vi "导入Excel.vi"(8 "error in (no error)":errorcluster) -> (0 "error out":errorcluster, 3 "data":string[][](array[string]))   [LabVIEW 2016, in "Alarm interface.lvlib"]
uses:
  Alarm interface.lvlib
  <vilib>/addons/_office/excel.llb/Excel Get Data ([str]).vi
  <vilib>/regexp/Match Regular Expression.xnode
  <vilib>/Utility/NIReport.llb/NI_report.lvclass
  <vilib>/Utility/NIReport.llb/Excel/NI_Excel.lvclass
  <vilib>/addons/_office/NI_ReportGenerationToolkit.lvlib
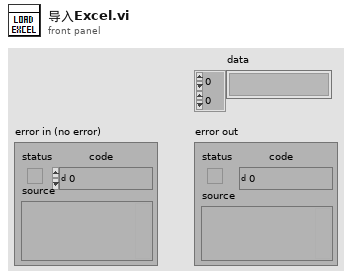
[diagram p1: front panel]
types:
  T1 = enum16{"Standard Report", "HTML", "Word", "Excel"}
  T2 = enum16{"maximized", "minimized", "normal", "no change"}
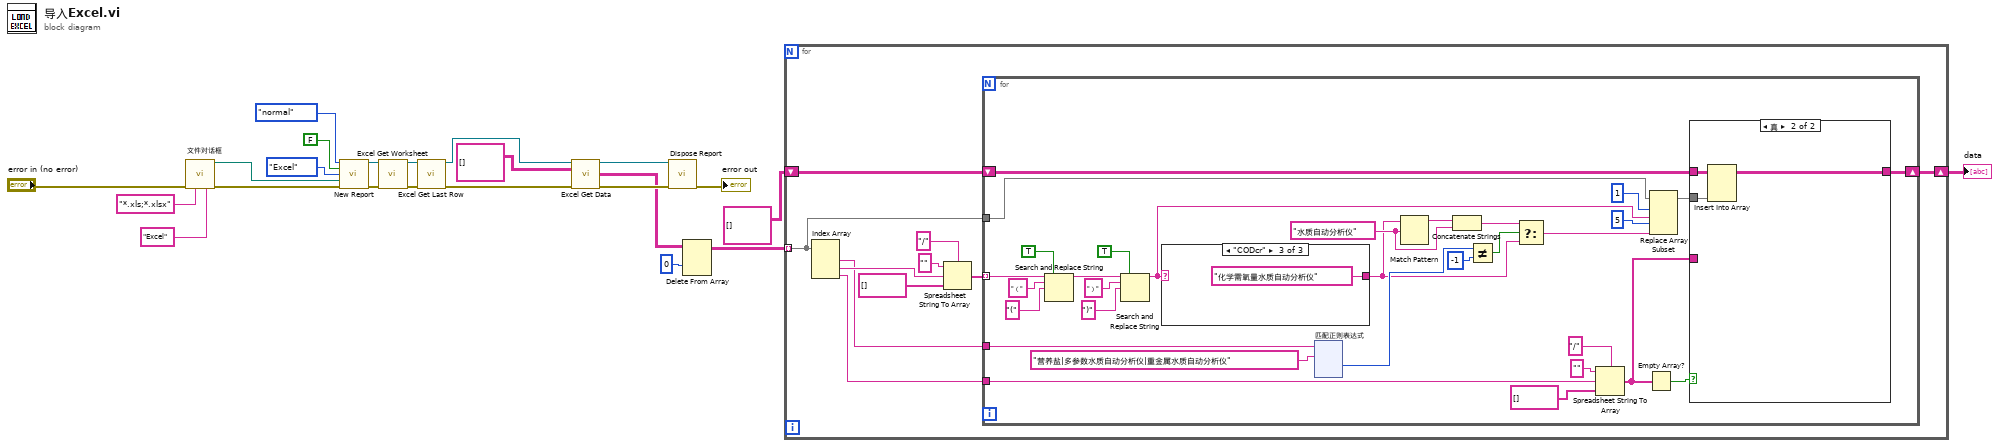
[diagram p0: block diagram]
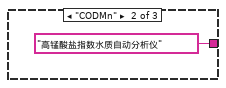
[diagram p3: hidden frame]
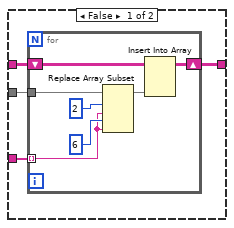
[diagram p4: hidden frame]
diagram:
  n1 = call "文件对话框"("error in"="error in (no error)", "pattern (all files)"="*.xls;*.xlsx" ("pattern label"), "pattern label"="Excel" ("pattern (all files)")) -> ("selected path"=w11:path, "error out"=w10:errorcluster)  [unwired: 9 in, 2 out]
  n2 = call <vilib>:"New Report.vi"("window state (normal)"=T2."normal", "display alerts? (F)"=FALSE, "report type"=T1."Excel", "template (empty)"=w11, "error in (no error)"=w10) -> ("report out"=w18:refnum<class "NI_report.lvclass">, "error out"=w12:errorcluster)  [unwired: 9 in]
  n3 = call <vilib>:"Excel Get Worksheet.vi"("report in"=w18, "error in (no error)"=w12) -> ("report out"=w23:refnum<class "NI_report.lvclass">, "error out"=w22:errorcluster)  [unwired: 12 in]
  n4 = call <vilib>:"Excel Get Last Row.vi"("report in"=w23, "error in (no error)"=w22) -> ("report out"=w21:refnum<class "NI_report.lvclass">, "error out"=w20:errorcluster)  [unwired: 11 in, 1 out]
  n5 = call-poly <vilib>:"Excel Get Data.vi"("report in"=w21, "data type"=string[][] [], "error in (no error)"=w20) -> ("report out"=w17:refnum<class "NI_report.lvclass">, "data"=w6:string[][], "error out"=w16:errorcluster)  [unwired: 10 in]
  n6 = call-dynamic "Dispose Report.vi"("report in"=w17, "error in (no error)"=w16) -> ("error out"=→"error out":errorcluster)  [unwired: 13 in]
  n7 = Delete From Array(array=w6, index (row)=0 ("索引 (行)")) -> (array with subset deleted=w7:string[][])  [unwired: 2 in, 1 out]
  n8 = for {
    tunnel: w7 -> [w30] mode=indexing
    shift-right: [w24] -> w2
    shift-left: string[][] [] ("data") -> [w25]
    n9 = Index Array(array=w30) -> (element #1=w27:string, element #2=w29:string, element #3=w28:string)  [unwired: 3 in]
    n10 = Spreadsheet String To Array(delimiter (Tab)="/" ("分隔符(Tab)"), format string="" ("格式字符串"), spreadsheet string=w29, array type (2D Dbl)=string[] []) -> (array=w26:string[])
    n11 = for {
      tunnel: w26 -> [w42] mode=indexing
      tunnel: w30 -> [w64]
      shift-right: [w44] -> w24
      shift-left: w25 -> [w45]
      tunnel: w28 -> [w53]
      tunnel: w27 -> [w49]
      w59 = "水质自动分析仪" ("正则表达式")
      n12 = Search and Replace String(replace all?=TRUE ("替换全部？(F)"), input string=w42, search string="（" ("搜索字符串"), replace string="(" ("搜索字符串")) -> (result string=w39:string)  [unwired: 4 in, 3 out]
      n13 = Search and Replace String(replace all?=TRUE ("替换全部？(F)"), input string=w39, search string="）" ("搜索字符串"), replace string=")" ("替换字符串(\"\")")) -> (result string=w38:string)  [unwired: 4 in, 3 out]
      n14 = case shown="\"CODcr\"" w38 {
        selector: w38 -> [w65 _ _]
        tunnel: [w65 "高锰酸盐指数水质自动分析仪" ("正则表达式") "化学需氧量水质自动分析仪" ("正则表达式")] -> w43
        frame Default {
        }
        frame "CODMn" {
        }
        frame "CODcr" {
        }
      }
      n15 = xnode "匹配正则表达式"("输入字符串"=w49, "正则表达式"="营养盐|多参数水质自动分析仪|重金属水质自动分析仪") -> ("匹配后偏移量"=w52:i32)  [unwired: 4 in, 4 out]
      n16 = Match Pattern(string=w43, regular expression=w59) -> (before substring=w60:string)  [unwired: 1 in, 3 out]
      n17 = Concatenate Strings(w60, w59) -> (w58:string)
      n18 = Not Equal?(x=w52, y=-1) -> (x != y?=w48:bool)
      n19 = Select(t=w58, s=w48, f=w43) -> (s? t:f=w61:string)
      n20 = Spreadsheet String To Array(delimiter (Tab)="/" ("分隔符(Tab)"), format string="" ("格式字符串"), spreadsheet string=w53, array type (2D Dbl)=string[] []) -> (array=w47:string[])
      n21 = Empty Array?(array=w47) -> (empty?=w46:bool)
      n22 = Replace Array Subset(array=w64, new element #1=w38, index #1=1 ("索引"), new element #2=w61, index #2=5 ("索引")) -> (w57:string[])
      n23 = case shown="真" w46 {
        tunnel: w57 -> [w71 w79]
        tunnel: [w70 w80] -> w44
        tunnel: w47 -> [w69 _]
        tunnel: w45 -> [w68 w81]
        frame False {
          n24 = for {
            tunnel: w71 -> [w78]
            tunnel: w69 -> [w75] mode=indexing
            shift-right: [w72] -> w70
            shift-left: w68 -> [w74]
            n25 = Replace Array Subset(array=w78, new element #1=w75, index #1=2 ("索引"), new element #2=w75, index #2=6 ("索引")) -> (w73:string[])
            n26 = Insert Into Array(array=w74, new element=w73) -> (w72:string[][])  [unwired: 2 in]
          }
        }
        frame True {
          n27 = Insert Into Array(array=w81, new element=w79) -> (w80:string[][])  [unwired: 2 in]
        }
      }
    }
  }
  "data" <- w2
